vi "shutter-control-reset.vi"(8 "error in":errorcluster, 11 "reference":refnum<vi>) -> (0 "error out":errorcluster)   [LabVIEW 2014]
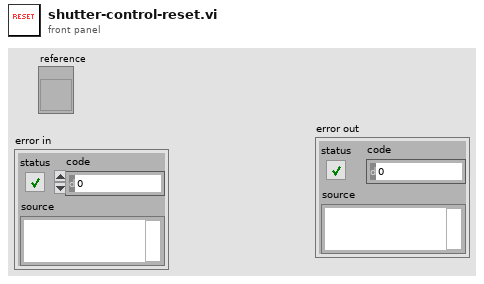
[diagram p1: front panel]
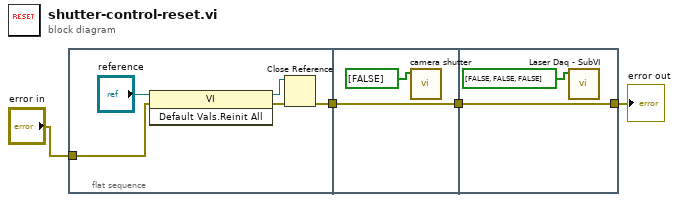
[diagram p0: block diagram]
diagram:
  n1 = flat-sequence {
    tunnel: [w7] -> w4
    tunnel: "error in" -> [w6]
    tunnel: w4 -> [w11]
    tunnel: [w11] -> w3
    tunnel: [w13] -> w2
    tunnel: w3 -> [w13]
    frame #0 {
      n2 = invoke class="VI" method="Default Vals.Reinit All"(reference="reference", error in=w6) -> (reference out=w9:refnum<vi>, error out=w8:errorcluster)  [unwired: 1 in, 1 out]
      n3 = Close Reference(reference=w9, error in (no error)=w8) -> (error out=w7:errorcluster)
    }
    frame #1 {
      n4 = call "camera shutter.vi"("Camera Input Switch"=bool[] [FALSE]) -> ()  [unwired: 10 in, 1 out]
    }
    frame #2 {
      n5 = call "Laser Daq - SubVI.vi"("Array"=bool[] [FALSE, FALSE, FALSE]) -> ()  [unwired: 11 in]
    }
  }
  "error out" <- w2
